vi "Initial, set and read, loop, pause (20190221).vi"() -> ()   [LabVIEW 2017]
panel:
  out "Wavelength Set":bool=TRUE
  out "Current Wavelength":dbl
  out "Output Wavelength":dbl
  out "error out 2":errorcluster
  out "State of Mono_SetWavelength":bool=TRUE
  out "Paused":bool
  in  "Pause Request":bool
  out "Total points":i32=5
  out "WL Range":dbl[](array[numeric])=[800.0, 850.0, 900.0, 950.0, 1000.0]
  in  "Step size (nm)":sgl=50.0 min=1 step=0.1
  in  "End Wavelength (nm)":dbl=1300.0 min=250.0 max=1350.0 step=0.1
  in  "Start Wavelength (nm)":dbl=500.0 min=250.0 max=1200.0 step=0.1
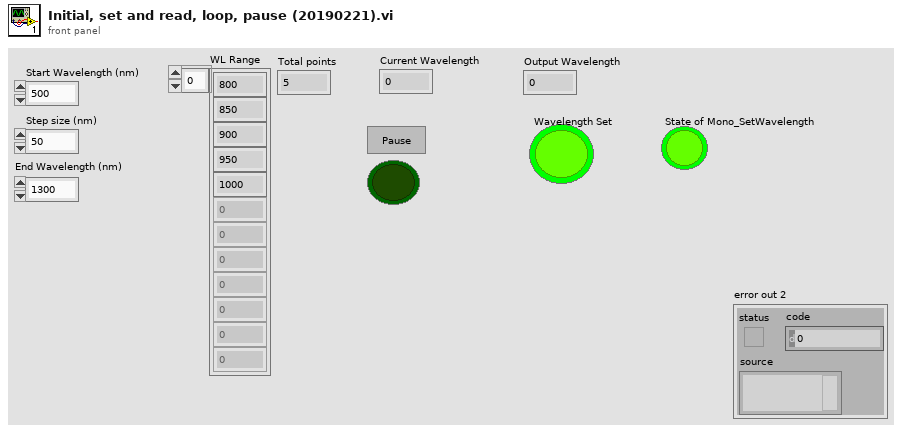
[diagram p1: front panel]
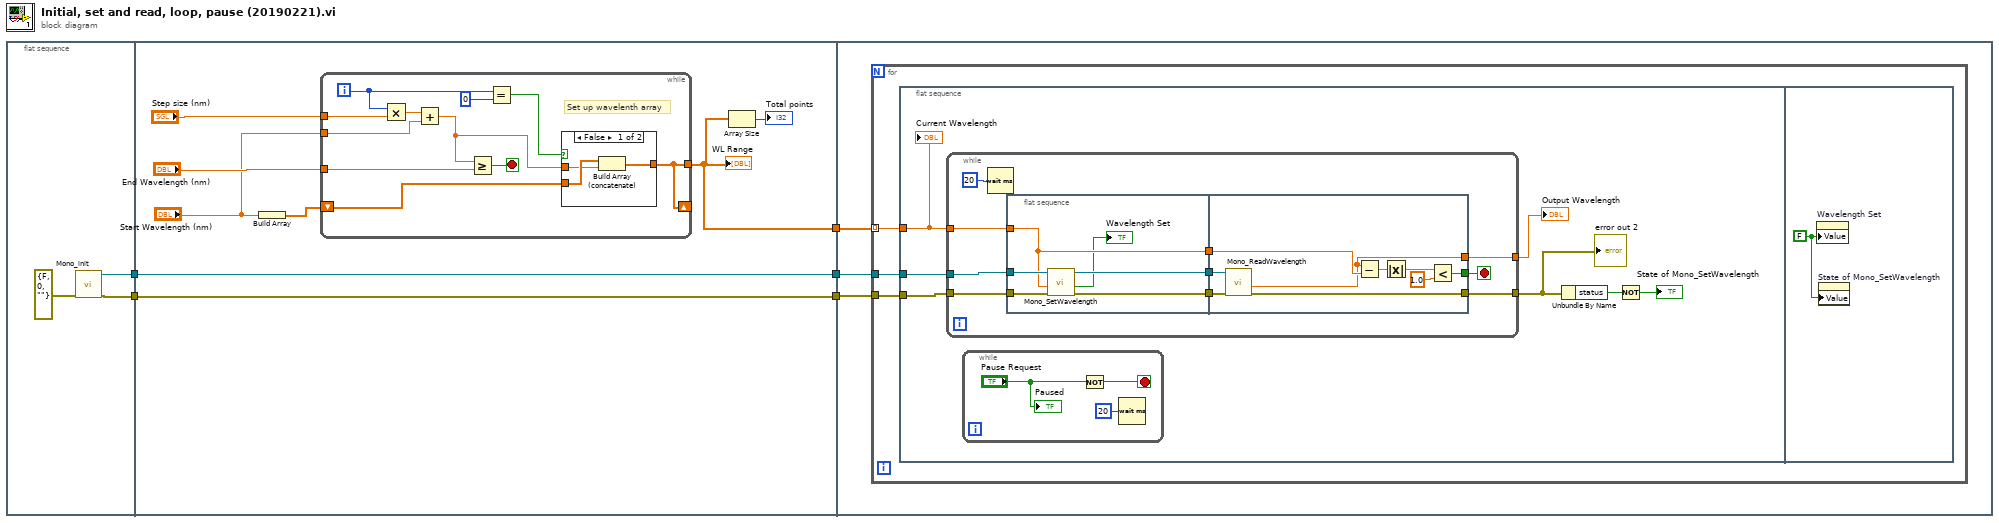
[diagram p0: block diagram]
diagram:
  n1 = flat-sequence {
    tunnel: [w7] -> w5
    tunnel: [w6] -> w3
    tunnel: w5 -> [w16]
    tunnel: [w16] -> w4
    tunnel: w3 -> [w15]
    tunnel: [w15] -> w2
    tunnel: [w10] -> w1
    tunnel: w4 -> [w34]
    tunnel: w2 -> [w33]
    tunnel: w1 -> [w32]
    frame #0 {
      n2 = call "Mono_init.vi"("error in (no error)"=errorcluster {"status"=FALSE, "code"=0, "source"=""}) -> ("error out"=w7:errorcluster, "CmdLib"=w6:refnum<k24>)  [unwired: 8 in, 1 out]
    }
    frame #1 {
      n3 = Build Array "Build Array"("Start Wavelength (nm)") -> (w11:dbl[])
      n4 = while {
        shift-right: [w17] -> _
        shift-left: w11 -> [w19]
        tunnel: "Step size (nm)" -> [w26]
        tunnel: "End Wavelength (nm)" -> [w27]
        tunnel: "Start Wavelength (nm)" -> [w20]
        tunnel: [w17] -> w10
        i -> [w22]
        stop <- w24 stop-if-true
        # "Set up wavelenth array"
        n5 = Multiply(x=w22, y=w26) -> (x*y=w25:sgl)
        n6 = Add(x=w25, y=w20) -> (x+y=w18:dbl)
        n7 = Greater Or Equal?(x=w18, y=w27) -> (x >= y?=w24:bool)
        n8 = Equal?(x=w22, y=0) -> (x = y?=w21:bool)
        n9 = case shown="False" w21 {
          tunnel: w19 -> [w30 w31]
          tunnel: w18 -> [w29 _]
          tunnel: [w28 w31] -> w17
          frame False {
            n10 = Build Array (concatenate)(w30, w29) -> (w28:dbl[])
          }
          frame True {
          }
        }
      }
      "WL Range" <- w10
      n11 = Array Size(array=w10) -> (size(s)=→"Total points":i32)
    }
    frame #2 {
      n12 = for {
        tunnel: w34 -> [w35]
        tunnel: w33 -> [w36]
        tunnel: w32 -> [w37] mode=indexing
        n13 = flat-sequence {
          tunnel: w35 -> [w38]
          tunnel: w36 -> [w40]
          tunnel: w37 -> [w39]
          frame #0 {
            n14 = while {
              tunnel: w38 -> [w49]
              tunnel: w40 -> [w48]
              tunnel: [w47] -> w41
              tunnel: [w46] -> w44
              tunnel: w39 -> [w45]
              stop <- w51 stop-if-true
              n15 = Wait (ms)(milliseconds to wait=u32 20) -> ()  [unwired: 1 out]
              n16 = flat-sequence {
                tunnel: [w59] -> w54
                tunnel: [w58] -> w53
                tunnel: [w56] -> w52
                tunnel: w49 -> [w60]
                tunnel: w48 -> [w57]
                tunnel: w45 -> [w56]
                tunnel: w54 -> [w68]
                tunnel: w53 -> [w69]
                tunnel: w52 -> [w67]
                tunnel: [w63] -> w51
                tunnel: [w62] -> w47
                tunnel: [w61] -> w46
                frame #0 {
                  n17 = call "Mono_SetWavelength.vi"("error in (no error) 2"=w60, "Wavelength"=w56, "CmdLib In"=w57) -> ("error out 2"=w59:errorcluster, "Wavelength Set"=→"Wavelength Set":bool, "CmdLib Out"=w58:refnum<k24>)  [unwired: 6 in]
                }
                frame #1 {
                  n18 = call "Mono_ReadWavelength.vi"("error in (no error) 2"=w68, "CmdLib In"=w69) -> ("error out 2"=w62:errorcluster, "getWavelength"=w61:dbl)  [unwired: 7 in, 1 out]
                  n19 = Subtract(x=w61, y=w67) -> (x-y=w66:dbl)
                  n20 = Absolute Value(x=w66) -> (abs(x)=w65:dbl)
                  n21 = Less?(x=w65, y=1.0) -> (x < y?=w63:bool)
                }
              }
            }
            "error out 2" <- w41
            "Output Wavelength" <- w44
            n22 = while {
              stop <- w71 stop-if-true
              n23 = Not(x="Pause Request") -> (.not. x?=w71:bool)
              n24 = Wait (ms)(milliseconds to wait=u32 20) -> ()  [unwired: 1 out]
              "Paused" <- "Pause Request"
            }
            n25 = Unbundle By Name(w41) -> ("status"=w42:bool)
            n26 = Not(x=w42) -> (.not. x?=→"State of Mono_SetWavelength":bool)
            "Current Wavelength" <- w39
          }
          frame #1 {
            w73 = FALSE ("Wavelength Set")
            n27 = property on="Wavelength Set" class="Bool (strict)"("Value"=w73) -> ()  [unwired: 2 in, 2 out]
            n28 = property on="State of Mono_SetWavelength" class="Bool (strict)"("Value"=w73) -> ()  [unwired: 2 in, 2 out]
          }
        }
      }
    }
  }
